vi "RestartPico.vi"(8 "Which Button?":T1(ring), 11 "Tn":timestamp) -> ()   [LabVIEW 2025]
uses:
  Globals.vi
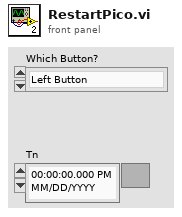
[diagram p1: front panel]
types:
  T1 = enum16{"Left Button", "Center Button", "Right Button", "Window Close"}
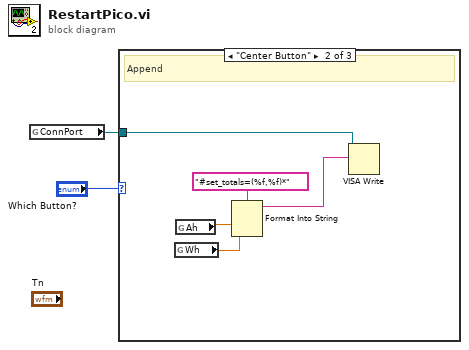
[diagram p0: block diagram]
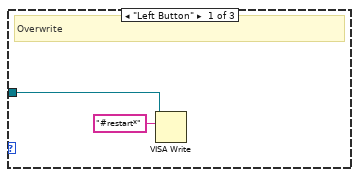
[diagram p2: hidden frame]
diagram:
  n1 = global read "Globals.vi" "ConnPort"() -> (w1:refnum<visa-resource-name>)
  n2 = case shown="\"Center Button\"" "Which Button?" {
    tunnel: w1 -> [w4 w6 _]
    frame "Left Button" {
      # "Overwrite"
      n3 = VISA Write(VISA resource name=w4, write buffer="#restart*") -> ()  [unwired: 1 in, 3 out]
    }
    frame "Center Button" {
      # "Append"
      n4 = global read "Globals.vi" "Wh"() -> (w7:dbl)
      n5 = global read "Globals.vi" "Ah"() -> (w8:dbl)
      n6 = Format Into String(format string="#set_totals=(%f,%f)*", w8, w7) -> (resulting string=w5:string)  [unwired: 2 in, 1 out]
      n7 = VISA Write(VISA resource name=w6, write buffer=w5) -> ()  [unwired: 1 in, 3 out]
    }
    frame "Right Button", Default {
      # "Cancel"
    }
  }
